vi "GPIO_Setup (SubVI).vi"(8 "error in (no error)":errorcluster, 9 "Pin Mode":bool[](array[boolean]), 10 "GPIO":bool[](array[boolean]), 11 "VISA resource name":refnum<visa-resource-name>) -> (0 "error out":errorcluster, 3 "VISA resource name out":refnum<visa-resource-name>)   [LabVIEW 2018]
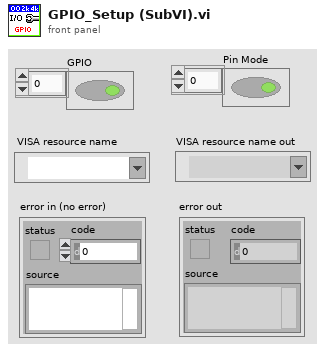
[diagram p1: front panel]
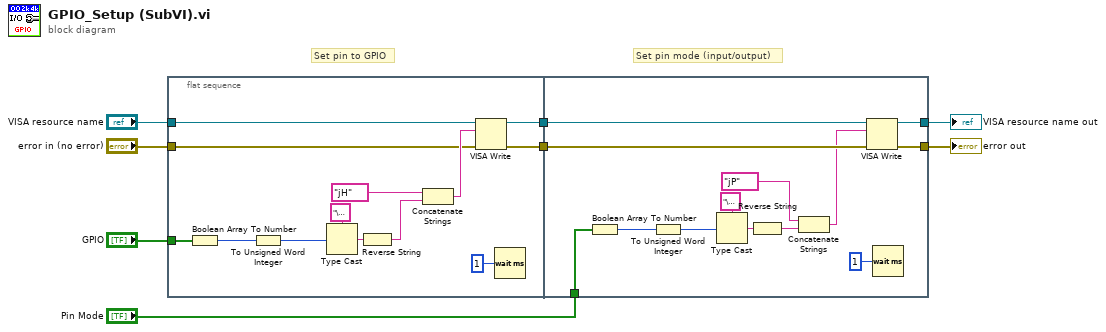
[diagram p0: block diagram]
diagram:
  # "Set pin to GPIO"
  # "Set pin mode (input/output)"
  n1 = flat-sequence {
    tunnel: [w16] -> w8
    tunnel: [w15] -> w7
    tunnel: "VISA resource name" -> [w14]
    tunnel: "error in (no error)" -> [w13]
    tunnel: "GPIO" -> [w9]
    tunnel: w8 -> [w30]
    tunnel: w7 -> [w29]
    tunnel: [w28] -> w4
    tunnel: [w27] -> w3
    tunnel: "Pin Mode" -> [w23]
    frame #0 {
      n2 = Boolean Array To Number(Boolean array=w9) -> (number=w11:u32)
      n3 = To Unsigned Word Integer(number=w11) -> (unsigned 16bit integer=w10:u16)
      n4 = Type Cast(type="\u0000", x=w10) -> (*(type *) &x=w20:string)
      n5 = Reverse String(1:w20) -> (0:w21:string)
      n6 = Concatenate Strings("jH" ("string"), w21) -> (w17:string)
      n7 = VISA Write(VISA resource name=w14, write buffer=w17, error in (no error)=w13) -> (VISA resource name out=w16:refnum<visa-resource-name>, error out=w15:errorcluster)  [unwired: 1 out]
      n8 = Wait (ms)(milliseconds to wait=u32 1) -> ()  [unwired: 1 out]
    }
    frame #1 {
      n9 = Boolean Array To Number(Boolean array=w23) -> (number=w24:u32)
      n10 = To Unsigned Word Integer(number=w24) -> (unsigned 16bit integer=w22:u16)
      n11 = Type Cast(type="\u0000", x=w22) -> (*(type *) &x=w33:string)
      n12 = Reverse String(1:w33) -> (0:w34:string)
      n13 = Concatenate Strings("jP" ("string"), w34) -> (w25:string)
      n14 = VISA Write(VISA resource name=w30, write buffer=w25, error in (no error)=w29) -> (VISA resource name out=w28:refnum<visa-resource-name>, error out=w27:errorcluster)  [unwired: 1 out]
      n15 = Wait (ms)(milliseconds to wait=u32 1) -> ()  [unwired: 1 out]
    }
  }
  "VISA resource name out" <- w4
  "error out" <- w3
